vi "SetSourceFunction.vi"(7 "SMU":T2, 8 "Error In":errorcluster, 10 "Source Function":T1, 11 "Keithley 2602 In":refnum<visa-resource-name>) -> (0 "Error Out":errorcluster, 3 "Keithley 2602 Out":refnum<visa-resource-name>)   [LabVIEW 2013, in "Keithley-2602.lvlib"]
uses:
  Keithley-2602.lvlib
  Controls/SMU.ctl
  Controls/SourceFunction.ctl
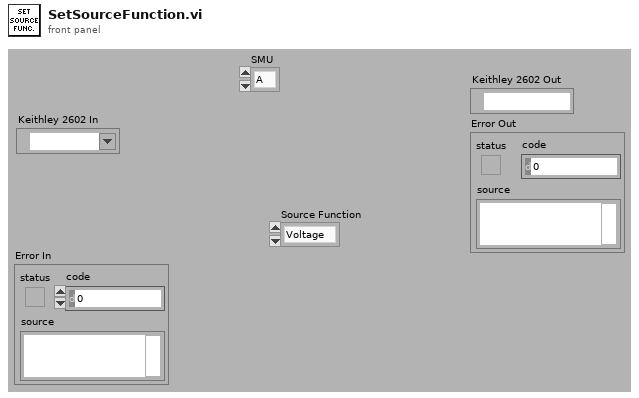
[diagram p1: front panel]
types:
  T1 = typedef "Keithley-2602.lvlib/SourceFunction.ctl" = enum16{"Voltage", "Current"}
  T2 = typedef "Keithley-2602.lvlib/SMU.ctl" = enum16{"A", "B"}
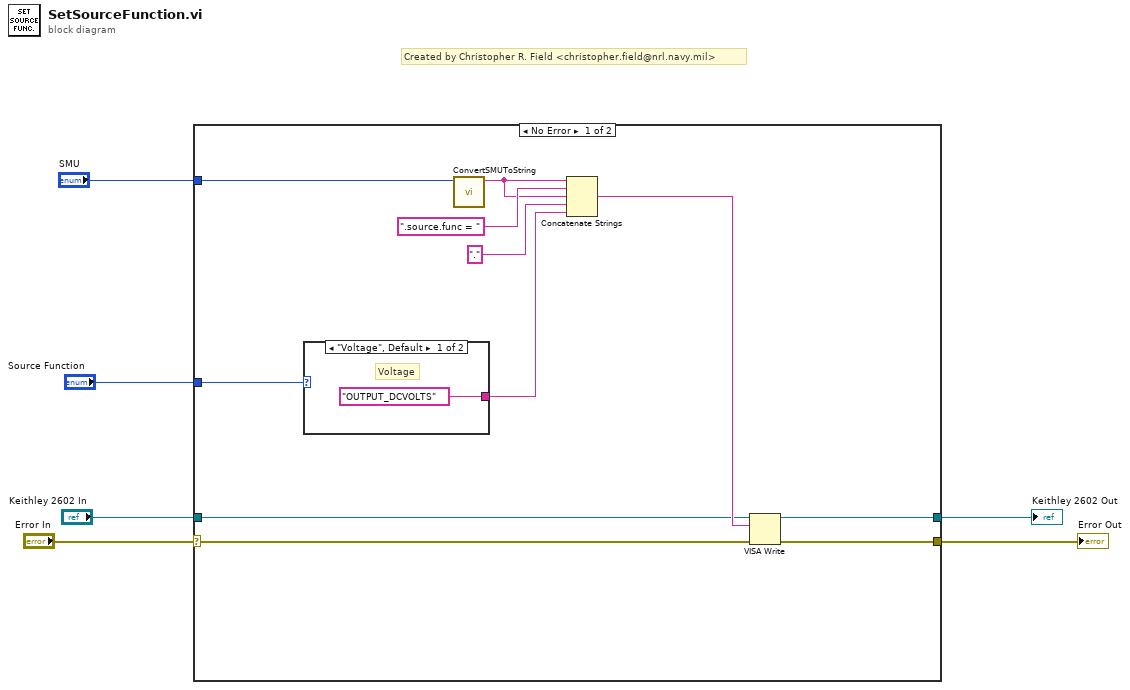
[diagram p0: block diagram]
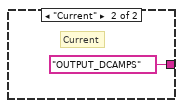
[diagram p2: hidden frame]
diagram:
  # "Created by Christopher R. Field <christopher.field@nrl.navy.mil>"
  n1 = case shown="No Error" "Error In" {
    selector: "Error In" -> [w7 w20]
    tunnel: "Keithley 2602 In" -> [w15 w21]
    tunnel: [w14 w21] -> w5
    tunnel: [w13 w20] -> w4
    tunnel: "SMU" -> [w9 _]
    tunnel: "Source Function" -> [w8 _]
    frame No Error {
      n2 = case shown="\"Voltage\", Default" w8 {
        tunnel: ["OUTPUT_DCVOLTS" "OUTPUT_DCAMPS"] -> w10
        frame "Voltage", Default {
          # "Voltage"
        }
        frame "Current" {
          # "Current"
        }
      }
      n3 = call "ConvertSMUToString.vi"("SMU"=w9) -> ("Channel"=w12:string)  [unwired: 10 in]
      n4 = Concatenate Strings(w12, ".source.func = ", w12, "." ("string"), w10) -> (w16:string)
      n5 = VISA Write(VISA resource name=w15, write buffer=w16, error in (no error)=w7) -> (VISA resource name out=w14:refnum<visa-resource-name>, error out=w13:errorcluster)  [unwired: 1 out]
    }
    frame Error {
    }
  }
  "Keithley 2602 Out" <- w5
  "Error Out" <- w4
